vi "SUB_ReadCOM_NO_error.vi"(0 "error IO":errorcluster, 1 "VISA resource name":refnum<visa-resource-name>) -> (2 "error out":errorcluster, 4 "uart msg":string, 5 "VISA out":refnum<visa-resource-name>)   [LabVIEW 2011]
panel:
  out "status":bool
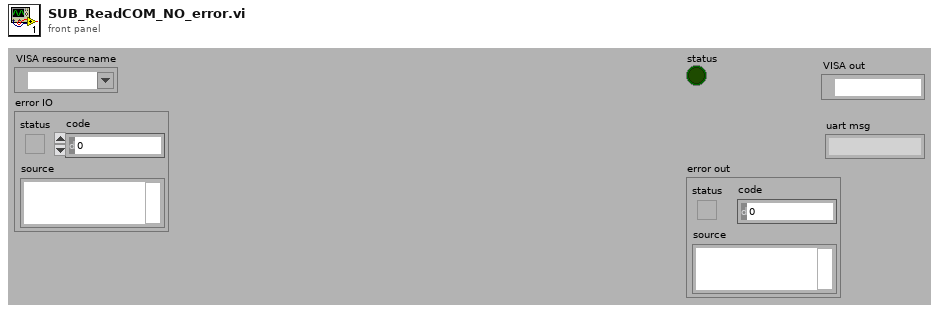
[diagram p1: front panel]
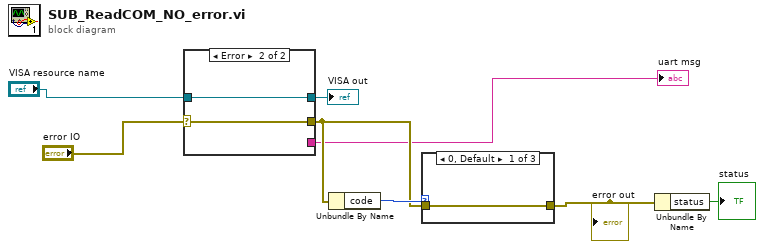
[diagram p0: block diagram]
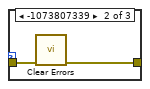
[diagram p2: hidden frame]
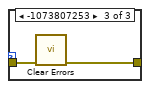
[diagram p3: hidden frame]
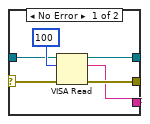
[diagram p4: hidden frame]
diagram:
  n1 = case "Read bytes from port." shown="Error" "error IO" {
    selector: "error IO" -> [w11 w16]
    tunnel: [w13 w16] -> w7
    tunnel: [w14 w15] -> w2
    tunnel: [w10 _] -> w3
    tunnel: "VISA resource name" -> [w9 w15]
    frame No Error {
      n2 = VISA Read(VISA resource name=w9, byte count=u32 100 ("bytes to read"), error in (no error)=w11) -> (VISA resource name out=w14:refnum<visa-resource-name>, read buffer=w10:string, error out=w13:errorcluster)  [unwired: 1 out]
    }
    frame Error {
      # "Error occurred \nreading Bytes at \nSerial Port"
    }
  }
  "uart msg" <- w3
  "VISA out" <- w2
  n3 = Unbundle By Name(w7) -> ("code"=w8:i32)
  n4 = case shown="0, Default" w8 {
    tunnel: w7 -> [w17 w19 w21]
    tunnel: [w17 w18 w20] -> w6
    frame 0, Default {
    }
    frame -1073807339 {
      n5 = call <vilib>:"Clear Errors.vi"("error in (no error)"=w19) -> ("error out"=w18:errorcluster)  [unwired: 6 in]
    }
    frame -1073807253 {
      n6 = call <vilib>:"Clear Errors.vi"("error in (no error)"=w21) -> ("error out"=w20:errorcluster)  [unwired: 6 in]
    }
  }
  "error out" <- w6
  n7 = Unbundle By Name(w6) -> ("status"=→"status":bool)
